vi "Point To Hub.vi"(10 "Current Heading":dbl) -> (1 "heading":dbl, 2 "omega":dbl format="%.2f")   [LabVIEW 2025]
uses:
  swerve-template/Type Definitions/Data/Robot Velocities.ctl
  <vilib>/Analysis/coordinate.llb/Angle Units.ctl
  <vilib>/Analysis/coordinate.llb/Angle Range (Degree).ctl
  <vilib>/Analysis/coordinate.llb/Wrap Angle (scalar).vi
  <vilib>/Rock Robotics/Network Tables/NT Read Numeric Array.vi
  Ballistic Utils/Get Distance LUT.vi
  <vilib>/addons/control/pid/pid.llb/PID (DBL).vi
  <vilib>/Analysis/NI_AAL_Angle.lvlib
  <vilib>/addons/control/pid/NI_PID_pid.lvlib
panel:
  in  "TOF LUT (s)":dbl[](array[numeric])
  in  "Input Velocities":T1
  in  "PID gains":T2={"proportional gain (Kc)"=1.0, "integral time (Ti, min)"=0.0, "derivative time (Td, min)"=0.0}
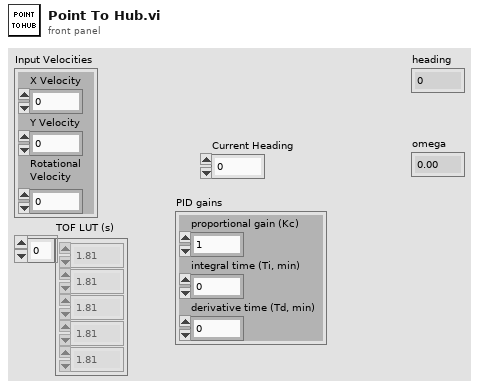
[diagram p1: front panel]
types:
  T1 = typedef "Robot Velocities.ctl" = cluster{"X Velocity":dbl, "Y Velocity":dbl, "Rotational \nVelocity":dbl}
  T2 = cluster{"proportional gain (Kc)":dbl, "integral time (Ti, min)":dbl, "derivative time (Td, min)":dbl}
  T3 = typedef "NI_AAL_Angle.lvlib/Angle Range (Degree).ctl" = u16
  T4 = typedef "NI_AAL_Angle.lvlib/Angle Units.ctl" = i32
  T5 = cluster{"Start Distance":i32, "Step Size":i32, "Max Distance":i32}
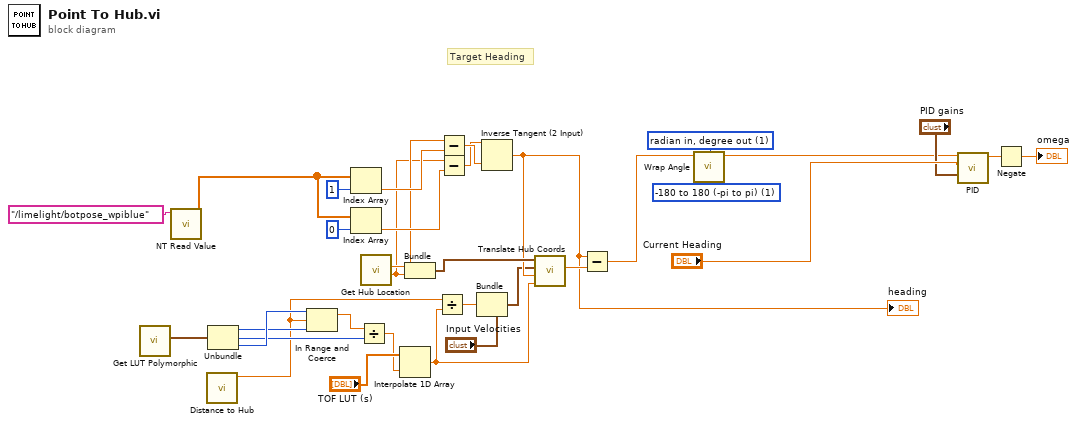
[diagram p0: block diagram]
diagram:
  w26 = T3 1 items=["none", "-180 to 180 (-pi to pi)", "0 to 360 (0 to 2pi)"] ("angle range")
  w27 = T4 1 items=["radian in, radian out", "radian in, degree out", "degree in, degree out", "degree in, radian out"] ("angle units")
  # "Target Heading"
  n1 = call-poly "Get LUT Polymorphic.vi"() -> ("Info"=w10:T5)  [unwired: 10 in, 1 out]
  n2 = call-poly <vilib>:"NT Read Value.vi"("name"="/limelight/botpose_wpiblue") -> ("value"=w30:dbl[])  [unwired: 8 in, 2 out]
  n3 = call "Distance to Hub.vi"() -> ("Distance to Hub (ft)"=w2:dbl)  [unwired: 10 in, 1 out]
  n4 = Unbundle(w10) -> ("Start Distance"=w8:i32, "Step Size"=w7:i32, "Max Distance"=w9:i32)
  n5 = In Range and Coerce(upper limit=w9, x=w2, lower limit=w8) -> (coerced(x)=w12:dbl)  [unwired: 1 out]
  n6 = Index Array(array=w30, index=1) -> (element=w31:dbl)
  n7 = Index Array(array=w30, index=0) -> (element=w28:dbl)
  n8 = Divide(x=w12, y=w7) -> (x/y=w11:dbl)
  n9 = call "Get Hub Location.vi"() -> ("Hub Y"=w16:dbl, "Hub X"=w17:dbl)  [unwired: 10 in]
  n10 = Interpolate 1D Array(1:w11, 2:"TOF LUT (s)") -> (0:w1:dbl)
  n11 = Bundle("Hub X"=w17, "Hub Y"=w16) -> (w18:cluster{"Hub X":dbl, "Hub Y":dbl})  [unwired: 1 in]
  n12 = Divide(x=w2, y=w1) -> (x/y=w4:dbl)
  n13 = Subtract(x=w17, y=w31) -> (x-y=w23:dbl)
  n14 = Subtract(x=w16, y=w28) -> (x-y=w22:dbl)
  n15 = Bundle(cluster="Input Velocities", "Y Velocity"=w4) -> (w3:T1)  [unwired: 2 in]
  n16 = Inverse Tangent (2 Input)(1:w23, 2:w22) -> (0:w6:dbl)
  "heading" <- w6
  n17 = call "Translate Hub Coords.vi"("TOF"=w1, "Point to Hub Theta"=w6, "Input Velocities"=w3, "Hub Coords"=w18) -> ("new theta"=w15:dbl)  [unwired: 5 in, 2 out]
  n18 = Subtract(x=w6, y=w15) -> (x-y=w14:dbl)
  n19 = call-poly <vilib>:"Wrap Angle.vi"("angle units"=w27, "angle range"=w26, "angle in"=w14) -> ("angle out"=w21:dbl)  [unwired: 7 in, 1 out]
  n20 = call-poly <vilib>:"PID.vi"("PID gains"="PID gains", "process variable"="Current Heading", "setpoint"=w21) -> ("output"=w20:dbl)  [unwired: 7 in, 1 out]
  n21 = Negate(x=w20) -> (-x=→"omega":dbl)
